vi "CalculateRsh.vi"(11 "Array":sgl[][](array[numeric])) -> (3 "Rsh (Ohm)":dbl)   [LabVIEW 2017]
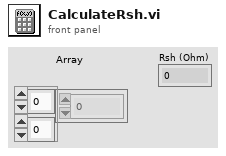
[diagram p1: front panel]
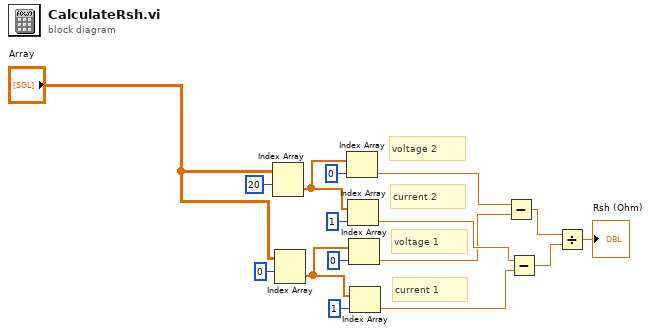
[diagram p0: block diagram]
diagram:
  # "current 1"
  # "voltage 1"
  # "current 2"
  # "voltage 2"
  n1 = Index Array(array="Array", index (row)=20) -> (element=w5:sgl[])  [unwired: 1 in]
  n2 = Index Array(array="Array", index (row)=0) -> (element=w8:sgl[])  [unwired: 1 in]
  n3 = Index Array(array=w5, index=0) -> (element=w12:sgl)
  n4 = Index Array(array=w5, index=1) -> (element=w14:sgl)
  n5 = Index Array(array=w8, index=0) -> (element=w13:sgl)
  n6 = Index Array(array=w8, index=1) -> (element=w15:sgl)
  n7 = Subtract(x=w12, y=w13) -> (x-y=w9:sgl)
  n8 = Subtract(x=w14, y=w15) -> (x-y=w10:sgl)
  n9 = Divide(x=w9, y=w10) -> (x/y=→"Rsh (Ohm)":sgl)
